vi "Helper-ConvertRelativeWaypointToReal.vi"(9 "Current boat location":T1 {"North" format="%#_10f"; "East" format="%#_8f"}, 10 "Relative Waypoints In":cluster{"X":dbl, "Y":dbl}[](array[cluster])) -> (1 "Actual Waypoints Out":refnum<class "Waypoint.lvclass">[](array[class]))   [LabVIEW 2013]
uses:
  Data/TypeDefs/UTM Location.ctl
  Classes/Waypoint/Waypoint.lvclass
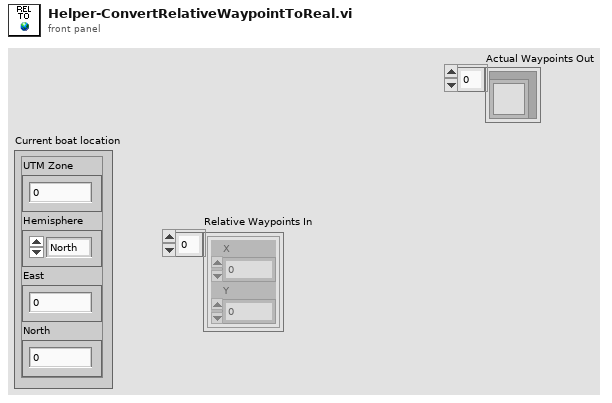
[diagram p1: front panel]
types:
  T1 = typedef "UTM Location.ctl" = cluster{"UTM Zone":dbl, "Hemisphere":enum16{"North", "South"}, "East":dbl, "North":dbl}
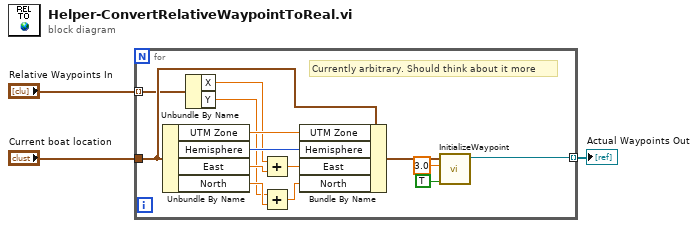
[diagram p0: block diagram]
diagram:
  n1 = for {
    tunnel: "Current boat location" -> [w15]
    tunnel: "Relative Waypoints In" -> [w10] mode=indexing
    tunnel: [w5] -> w1 mode=indexing
    # "Currently arbitrary. Should think about it more"
    n2 = Unbundle By Name(w15) -> ("UTM Zone"=w12:dbl, "Hemisphere"=w11:enum16{"North", "South"}, "East"=w17:dbl, "North"=w16:dbl)
    n3 = Unbundle By Name(w10) -> ("X"=w9:dbl, "Y"=w8:dbl)
    n4 = Add(x=w9, y=w17) -> (x+y=w14:dbl)
    n5 = Add(x=w8, y=w16) -> (x+y=w13:dbl)
    n6 = Bundle By Name(cluster=w15, "UTM Zone"=w12, "Hemisphere"=w11, "East"=w14, "North"=w13) -> (w7:T1)
    n7 = call "InitializeWaypoint.vi"("Sailing Point?"=TRUE, "Tolerance (meters?) (0)"=3.0, "Coords"=w7) -> ("Waypoint Out"=w5:refnum<class "Waypoint.lvclass">)  [unwired: 8 in]
  }
  "Actual Waypoints Out" <- w1
